vi "Query Current.vi"(8 "error in":errorcluster, 11 "ProXR in":refnum<class "ProXR.lvclass">) -> (0 "error out":errorcluster, 3 "ProXR out":refnum<class "ProXR.lvclass">)   [LabVIEW 2019, in "ProXR.lvlib" / "ProXR.lvclass"]
uses:
  Library/ProXR.lvclass
  Write Measured Current.vi
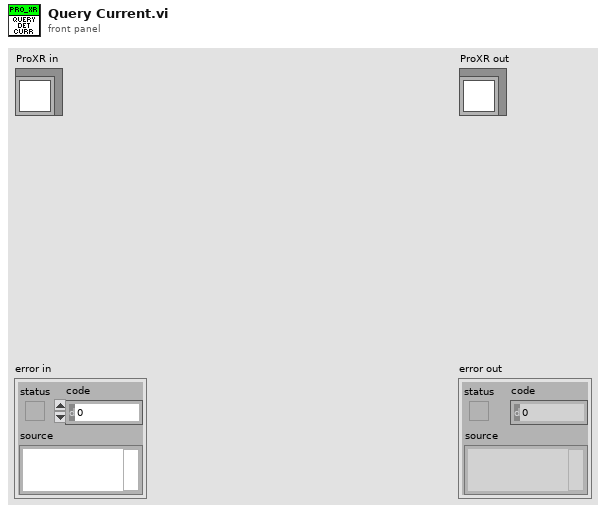
[diagram p1: front panel]
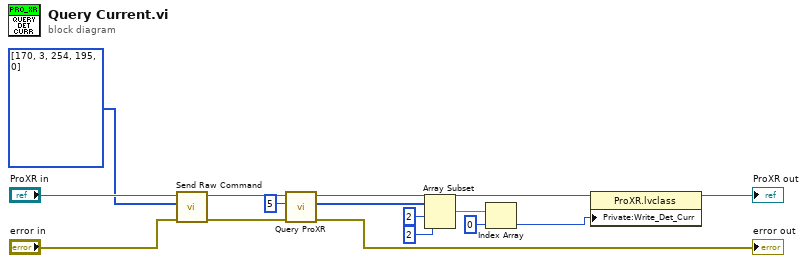
[diagram p0: block diagram]
diagram:
  n1 = call "Send Raw Command.vi"("error in"="error in", "Raw Command"=u8[] [170, 3, 254, 195, 0], "ProXR_IO in"="ProXR in") -> ("error out"=w13:errorcluster, "ProXR_IO out"=w12:refnum<class "ProXR.lvclass">)  [unwired: 7 in]
  n2 = call "Query ProXR.vi"("error in"=w13, "Bytes to Read"=u32 5, "ProXR_IO in"=w12) -> ("error out"=→"error out":errorcluster, "Response"=w9:u8[], "ProXR_IO out"=w4:refnum<class "ProXR.lvclass">)  [unwired: 6 in]
  n3 = Array Subset(array=w9, index=2, length=2) -> (w6:u8[])
  n4 = Index Array(array=w6, index=0) -> (element=w2:u8)
  n5 = property class="ProXR.lvclass"(reference=w4, "Private:Write_Det_Curr"=w2) -> (reference out=→"ProXR out":refnum<class "ProXR.lvclass">)  [unwired: 1 in, 1 out]
